vi "New Panel Reference.vi"(8 "error in (no error)":errorcluster, 10 "VI Refnum":refnum<vi>, 11 "Stage in":refnum<class "Stage.lvclass">) -> (0 "error out":errorcluster, 3 "Stage out":refnum<class "Stage.lvclass">)   [LabVIEW 2020, in "Stage.lvlib" / "Stage.lvclass"]
uses:
  Stage.lvclass
  C:/Program Files/National Instruments/LabVIEW 2020/vi.lib/ActorFramework/Actor/Actor.lvclass
  <vilib>/ActorFramework/Actor/Actor.lvclass/Actor.ctl
  Communication Messages/Send Panel Refercence Msg/Send Panel Refercence Msg.lvclass/Send Panel Refercence Msg.ctl
  <vilib>/ActorFramework/Message Enqueuer/Message Enqueuer.lvclass/Message Enqueuer.ctl
  <vilib>/ActorFramework/Message Enqueuer/Enqueue.vi
  Communication Messages/Send Panel Refercence Msg/Send Panel Refercence Msg.lvclass
  C:/Program Files/National Instruments/LabVIEW 2020/vi.lib/ActorFramework/Message/Message.lvclass
  <vilib>/ActorFramework/Message Priority Queue/Priority Enqueue.vi
  <vilib>/ActorFramework/Actor/Actor.lvclass
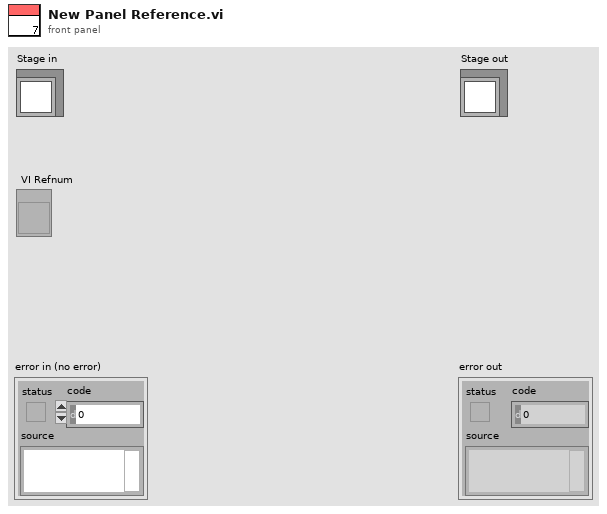
[diagram p1: front panel]
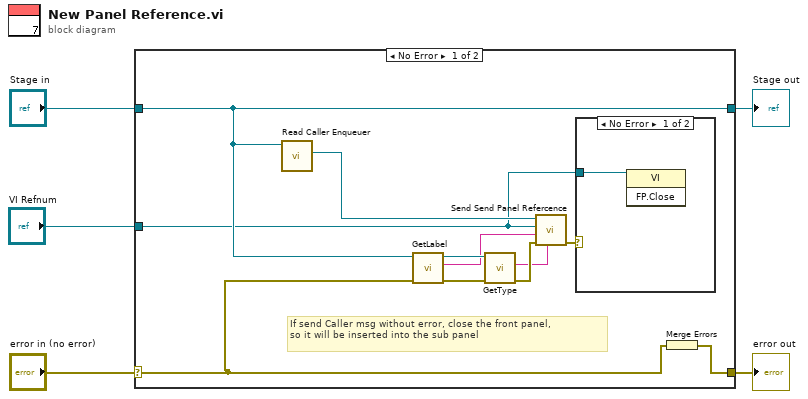
[diagram p0: block diagram]
diagram:
  n1 = case shown="No Error" "error in (no error)" {
    selector: "error in (no error)" -> [w15 w19]
    tunnel: [w14 w19] -> w4
    tunnel: [w16 w18] -> w2
    tunnel: "Stage in" -> [w16 w18]
    tunnel: "VI Refnum" -> [w6 _]
    frame No Error {
      # "If send Caller msg without error, close the front panel,\nso it will be inserted into the sub panel"
      n2 = call <vilib>:"Read Caller Enqueuer.vi"("Actor"=w16) -> ("Caller Enqueuer"=w8:refnum<class "Message Enqueuer.lvclass">)  [unwired: 10 in]
      n3 = call-dynamic "GetLabel.vi"("error in (no error)"=w15, "Device in"=w16) -> ("error out"=w13:errorcluster, "Label"=w10:string, "Device out"=w12:refnum<class "Stage.lvclass">)  [unwired: 7 in]
      n4 = call-dynamic "GetType.vi"("error in (no error)"=w13, "Device in"=w12) -> ("error out"=w11:errorcluster, "Type"=w9:string)  [unwired: 7 in, 1 out]
      n5 = call "Send Send Panel Refercence.vi"("Type"=w9, "error in (no error)"=w11, "Label"=w10, "VI Refnum"=w6, "Message Enqueuer"=w8) -> ("error out"=w7:errorcluster)  [unwired: 5 in, 1 out]
      n6 = case shown="No Error" w7 {
        tunnel: w6 -> [w17 _]
        frame No Error {
          n7 = invoke class="VI" method="FP.Close"(reference=w17) -> ()  [unwired: 2 in, 3 out]
        }
        frame Error {
        }
      }
      n8 = Merge Errors(w15) -> (w14:errorcluster)
    }
    frame Error {
    }
  }
  "error out" <- w4
  "Stage out" <- w2
